vi "Read Files.vi"(8 "error in (no error)":errorcluster, 11 "Masterv2 in":refnum<class "Masterv2.lvclass">) -> (0 "error out":errorcluster, 3 "Masterv2 out":refnum<class "Masterv2.lvclass">)   [LabVIEW 2014, in "Main Libraryv2.lvlib" / "Masterv2.lvclass"]
uses:
  Master/Masterv2.lvclass
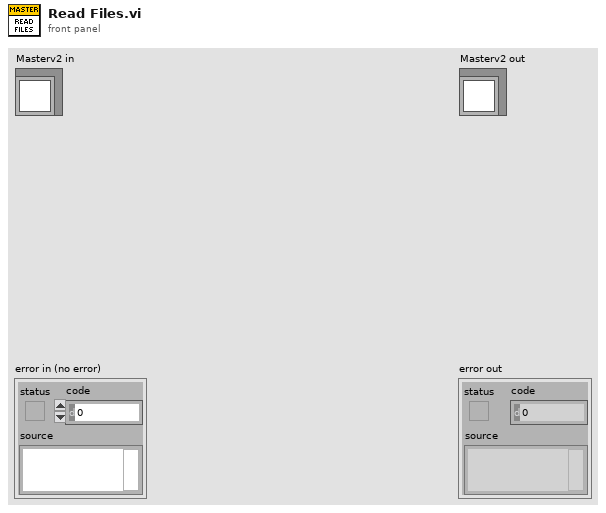
[diagram p1: front panel]
types:
  T1 = enum16{"open", "replace", "create", "open or create", "replace or create", "replace or create with confirmation"}
  T2 = cluster{"type string":i16[], "data string":string}
  T3 = cluster{"type string":i16[], "data string":string}[]
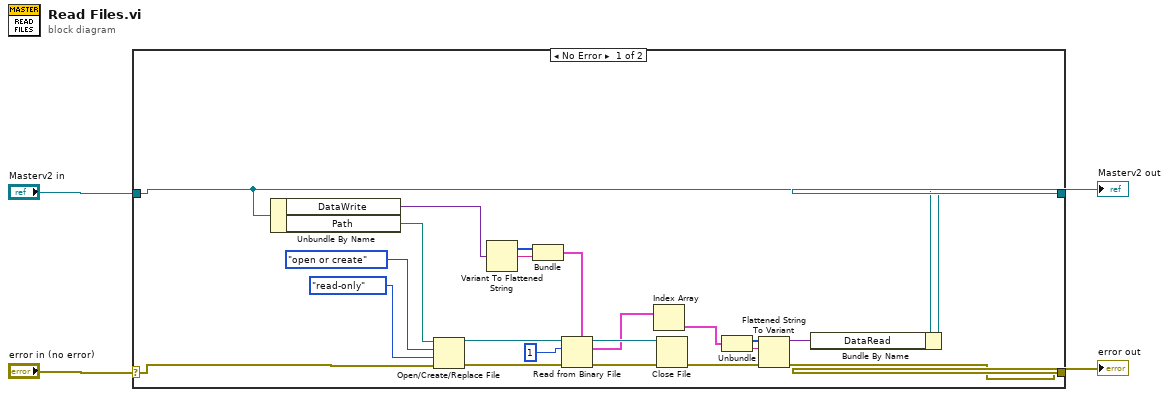
[diagram p0: block diagram]
diagram:
  n1 = case shown="No Error" "error in (no error)" {
    selector: "error in (no error)" -> [w7 w28]
    tunnel: [w8 w28] -> w3
    tunnel: [w6 w27] -> w1
    tunnel: "Masterv2 in" -> [w5 w27]
    frame No Error {
      n2 = Unbundle By Name(w5) -> ("DataWrite"=w9:variant, "Path"=w26:path)
      n3 = Open/Create/Replace File(file path (use dialog)=w26, error in=w7, operation (0:open)=T1."open or create", access (0:read/write)=enum16{"read/write", "read-only", "write-only"}."read-only") -> (refnum out=w23:refnum<file>, error out=w22:errorcluster)  [unwired: 2 in, 1 out]
      n4 = Variant To Flattened String(Variant=w9) -> (data string=w12:string, 1:w11:i16[])
      n5 = Bundle("type string"=w11, "data string"=w12) -> (w10:T2)  [unwired: 1 in]
      n6 = Read from Binary File(5:w10, 8:w22, 10:1 ("count (1)"), 11:w23) -> (0:w20:errorcluster, 2:w19:T3, 3:w21:refnum<file>)  [unwired: 2 in, 1 out]
      n7 = Index Array(array=w19) -> (element=w18:T2)  [unwired: 1 in]
      n8 = Close File(refnum=w21, error in=w20) -> (error out=w15:errorcluster)  [unwired: 1 out]
      n9 = Unbundle(w18) -> ("type string"=w17:i16[], "data string"=w16:string)
      n10 = Flattened String To Variant(4:w15, 6:w16, 7:w17) -> (0:w8:errorcluster, 3:w14:variant)
      n11 = Bundle By Name(cluster=w5, "DataRead"=w14) -> (w6:refnum<class "Masterv2.lvclass">)
    }
    frame Error {
    }
  }
  "error out" <- w3
  "Masterv2 out" <- w1
